vi "NPC3SG Convert Calibration v10.6.1.vi"(2 "Is Voltage?":bool, 3 "Axis":u16(ring) items=["X", "Y", "Z"], 4 "Input Value":dbl) -> (0 "Has calibration?":bool, 1 "Output Value":dbl)   [LabVIEW 2010]
uses:
  <vilib>/Utility/file.llb/Read From Spreadsheet File (DBL).vi
panel:
  out "Positions (µm)":dbl[](array[numeric])
  out "Voltages (V)":dbl[](array[numeric])
  in  "Config Name":string="NPC3SG Objective Calibration 220126"
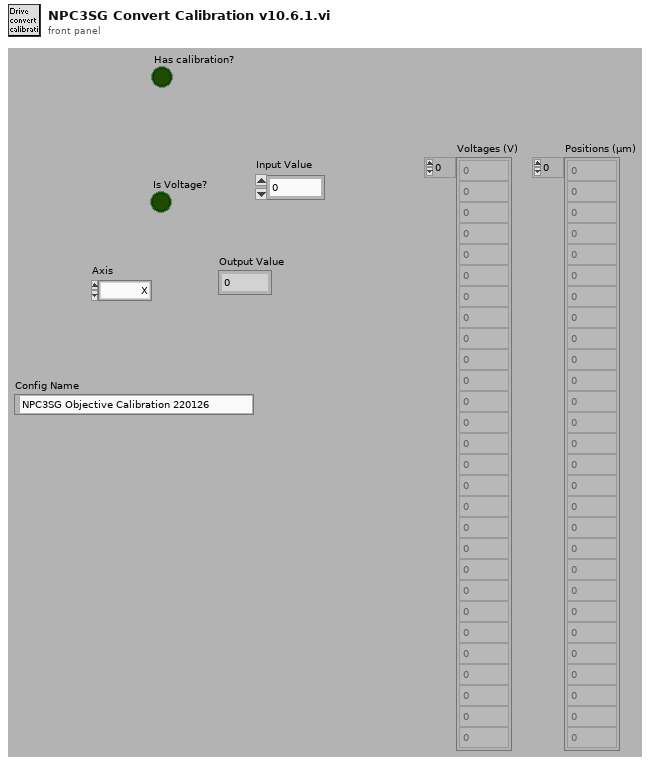
[diagram p1: front panel]
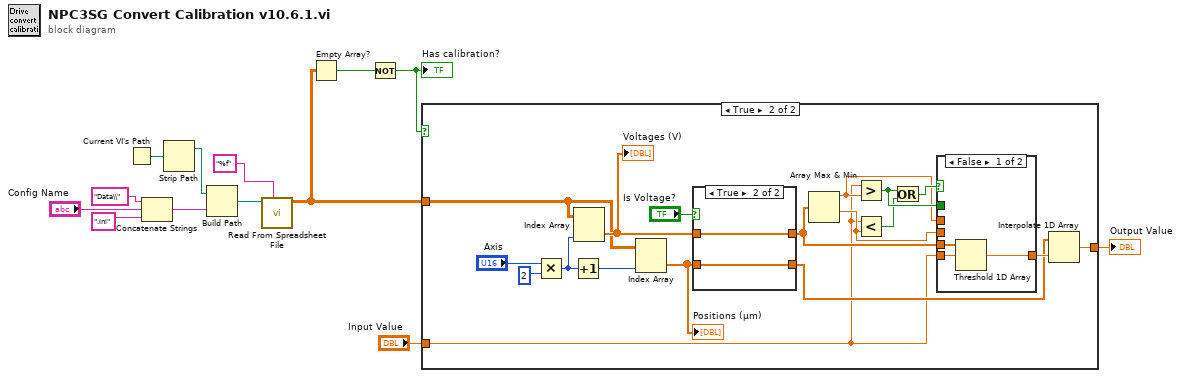
[diagram p0: block diagram]
diagram:
  n1 = Current VI's Path() -> (path=w9:path)
  n2 = Concatenate Strings("Data\\" ("name or relative path"), "Config Name", ".ini" ("name or relative path")) -> (w10:string)
  n3 = Strip Path(path=w9) -> (stripped path=w8:path)  [unwired: 1 out]
  n4 = Build Path(base path=w8, name or relative path=w10) -> (appended path=w7:path)
  n5 = call-poly <vilib>:"Read From Spreadsheet File.vi"("format (%.3f)"="%f", "file path (dialog if empty)"=w7) -> ("all rows"=w2:dbl[][])  [unwired: 5 in, 4 out]
  n6 = Empty Array?(array=w2) -> (empty?=w3:bool)
  n7 = Not(x=w3) -> (.not. x?=w1:bool)
  "Has calibration?" <- w1
  n8 = case shown="True" w1 {
    tunnel: [w14 w23] -> w5
    tunnel: "Input Value" -> [w14 w22]
    tunnel: w2 -> [_ w15]
    frame False {
    }
    frame True {
      n9 = Multiply(x="Axis", y=u16 2) -> (x*y=w21:u16)
      n10 = Increment(x=w21) -> (x+1=w20:u16)
      n11 = Index Array(array=w15, index (col)=w21) -> (element=w17:dbl[])  [unwired: 1 in]
      "Voltages (V)" <- w17
      n12 = Index Array(array=w15, index (col)=w20) -> (element=w16:dbl[])  [unwired: 1 in]
      "Positions (µm)" <- w16
      n13 = case shown="True" "Is Voltage?" {
        tunnel: [w42 w45] -> w32
        tunnel: w17 -> [w43 w45]
        tunnel: [w43 w44] -> w27
        tunnel: w16 -> [w42 w44]
        frame False {
        }
        frame True {
        }
      }
      n14 = Array Max & Min(array=w32) -> (max value=w25:dbl, min value=w24:dbl)  [unwired: 2 out]
      n15 = Greater?(x=w22, y=w25) -> (0:w30:bool)
      n16 = Less?(x=w22, y=w24) -> (x < y?=w28:bool)
      n17 = Or(x=w30, y=w28) -> (x .or. y?=w29:bool)
      n18 = case shown="False" w29 {
        tunnel: w30 -> [_ w39]
        tunnel: [w33 w38] -> w31
        tunnel: w32 -> [w35 _]
        tunnel: w22 -> [w34 _]
        tunnel: w25 -> [_ w37]
        tunnel: w24 -> [_ w36]
        frame False {
          n19 = Threshold 1D Array(2:w34, 3:w35) -> (0:w33:dbl)  [unwired: 1 in]
        }
        frame True {
          n20 = case shown="False" w39 {
            tunnel: [w40 w41] -> w38
            tunnel: w37 -> [_ w41]
            tunnel: w36 -> [w40 _]
            frame False {
            }
            frame True {
            }
          }
        }
      }
      n21 = Interpolate 1D Array(1:w31, 2:w27) -> (0:w23:dbl)
    }
  }
  "Output Value" <- w5
